vi "Test.vi"   [LabVIEW 2015]
uses:
  Initialize (Remote Device).vi
  SLSC Remote.lvclass
  SLSC Interface Class/SLSC Interface.lvclass
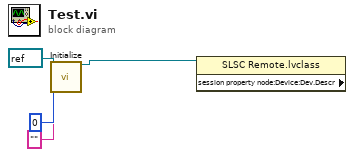
[diagram p0: block diagram]
diagram:
  n1 = call-poly "Initialize.vi"("devices"=refnum<k21> refnum, "Hostname/IP"="", "Port"=u16 0) -> ("SLSC Remote out"=w4:refnum<class "SLSC Remote.lvclass">)  [unwired: 11 in, 1 out]
  n2 = property class="SLSC Remote.lvclass" props=["session property node:Device:Dev.Descr"](reference=w4) -> ()  [unwired: 1 in, 3 out]
